vi "build_providers.vi"(8 "error in":errorcluster, 11 "path":path) -> (0 "error out":errorcluster, 3 "providers":refnum<class "system.logging.provider.lvclass">[](array[class]))   [LabVIEW 2021, in "system.logging.lvclass"]
uses:
  system.logging.lvclass
  system.logging.provider/system.logging.provider.lvclass
  configuration.ctl
  system.logging.provider/console.provider/console.provider.lvclass
  Z:/Projects/PCCS/labview-system-logging/source/system.logging.provider/system.logging.provider.lvclass
  system.logging.provider/json.provider/json.provider.lvclass
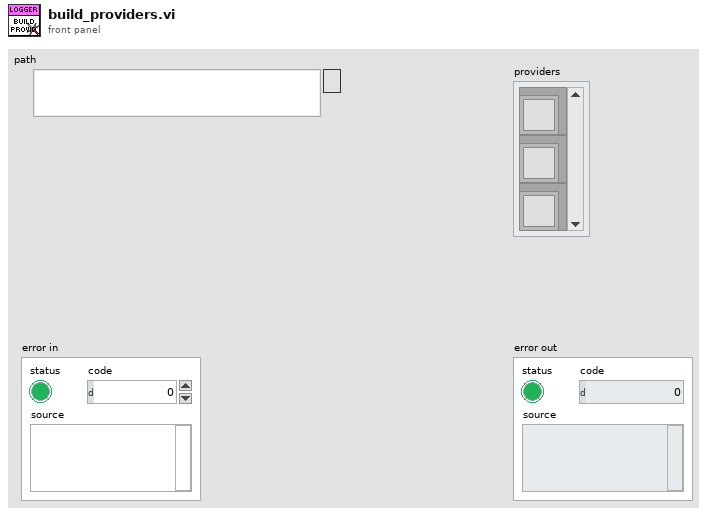
[diagram p1: front panel]
types:
  T1 = typedef "system.logging.lvclass/configuration.ctl" = cluster{"name":string, "enable":bool, "severity":string}
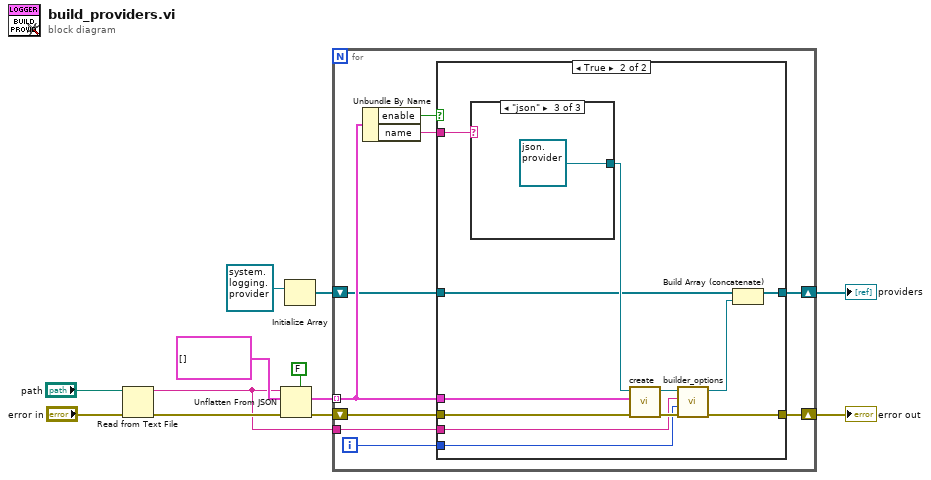
[diagram p0: block diagram]
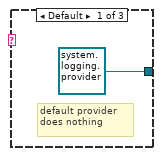
[diagram p3: hidden frame]
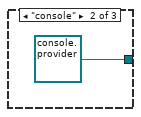
[diagram p4: hidden frame]
diagram:
  n1 = Read from Text File(file (use dialog)="path", error in="error in") -> (text=w1:string, error out=w10:errorcluster)  [unwired: 2 in, 2 out]
  n2 = Unflatten From JSON(enable LabVIEW extensions? (T)=FALSE, JSON string=w1, type and defaults=T1[] [], error in (no error)=w10) -> (value=w7:T1[], error out=w6:errorcluster)  [unwired: 3 in]
  n3 = Initialize Array(refnum<class "system.logging.provider.lvclass"> refnum ("system.logging.provider.lvclass")) -> (w2:refnum<class "system.logging.provider.lvclass">[])  [unwired: 1 in]
  n4 = for {
    tunnel: w7 -> [w17] mode=indexing
    shift-right: [w21] -> w5
    shift-left: w6 -> [w18]
    shift-right: [w19] -> w4
    shift-left: w2 -> [w15]
    tunnel: w1 -> [w14]
    i -> [w13]
    n5 = Unbundle By Name(w17) -> ("enable"=w16:bool, "name"=w20:string)
    n6 = case shown="True" w16 {
      tunnel: [w23 w28] -> w21
      tunnel: w20 -> [_ w35]
      tunnel: [w22 w30] -> w19
      tunnel: w18 -> [w23 w33]
      tunnel: w17 -> [_ w32]
      tunnel: w15 -> [w22 w31]
      tunnel: w14 -> [_ w25]
      tunnel: w13 -> [_ w24]
      frame False {
      }
      frame True {
        n7 = case shown="\"json\"" w35 {
          tunnel: [refnum<class "system.logging.provider.lvclass"> refnum ("system.logging.provider.lvclass") refnum<class "console.provider.lvclass"> refnum ("console.provider.lvclass") refnum<class "json.provider.lvclass"> refnum ("json.provider.lvclass")] -> w34
          frame Default {
            # "default provider\ndoes nothing"
          }
          frame "console" {
          }
          frame "json" {
          }
        }
        n8 = call-dynamic "create.vi"("error in (no error)"=w33, "configuration"=w32, "system.logging.provider in"=w34) -> ("error out"=w29:errorcluster, "system.logging.provider out"=w27:refnum<class "system.logging.provider.lvclass">)  [unwired: 7 in]
        n9 = call-dynamic "builder_options.vi"("error in (no error)"=w29, "path_index"=w24, "configuration"=w25, "system.logging.provider in"=w27) -> ("error out"=w28:errorcluster, "system.logging.provider out"=w26:refnum<class "system.logging.provider.lvclass">)  [unwired: 6 in]
        n10 = Build Array (concatenate)(w31, w26) -> (w30:refnum<class "system.logging.provider.lvclass">[])
      }
    }
  }
  "error out" <- w5
  "providers" <- w4
